vi "niFpgaFFTStreamingStateTransitionLogic.vi"(7 "reset":bool, 8 "output state in":enum8{"idle", "output"}(ring), 11 "process state in":enum8{"process", "idle"}(ring)) -> (0 "output state out":enum8{"idle", "output"}(ring), 2 "ready for input":bool, 3 "process state out":enum8{"process", "idle"}(ring))   [LabVIEW 2017]
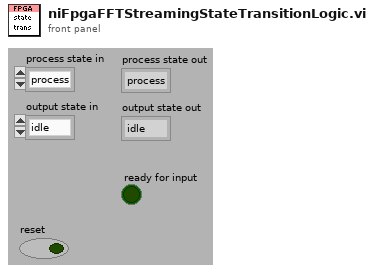
[diagram p1: front panel]
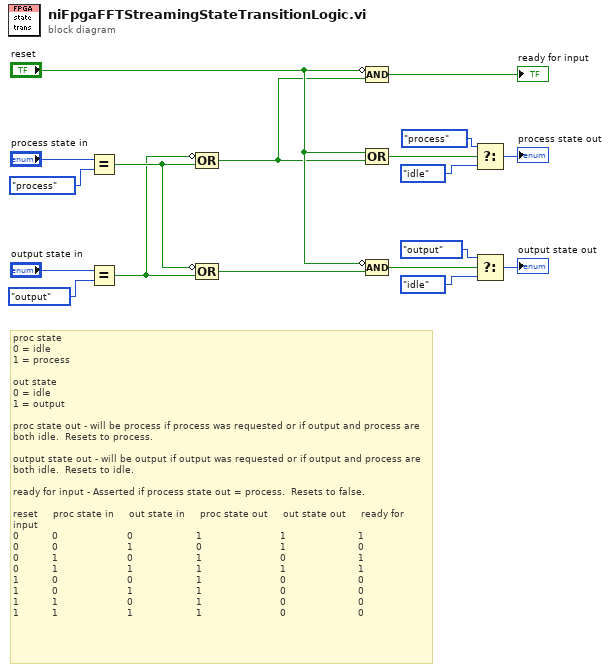
[diagram p0: block diagram]
diagram:
  # "proc state\n0 = idle\n1 = process\n\nout state\n0 = idle\n1 = output\n\nproc state out - will be process if process was requested or if output and process are both idle.  Resets to process.\n\noutput state out - will be output if output was requested or if output and process are both idle.  Resets to idle.\n\nready for input - Asserted if process state out = process.  Resets to false.\n\nreset     proc state in     out state in     proc state out     out state out     ready for input\n0           0                       0                     1                          1                        1 \n0           0                       1                     0                          1                        0\n0 \t\t        1                       0                     1                          0                        1\n0 \t\t        1                       1                     1                          1                        1\n1 \t\t        0                       0                     1                          0                        0\n1 \t\t        0                       1                     1                          0                        0\n1 \t\t        1                       0                     1                          0                        0\n1 \t\t        1                       1                     1                          0                        0"
  n1 = Equal?(x="process state in", y=enum8{"process", "idle"}."process") -> (x = y?=w5:bool)
  n2 = Equal?(x="output state in", y=enum8{"idle", "output"}."output" ("x")) -> (x = y?=w4:bool)
  n3 = Compound Arithmetic op=OR(invert w4, w5) -> (w3:bool)
  n4 = Compound Arithmetic op=OR(invert w5, w4) -> (w13:bool)
  n5 = Compound Arithmetic op=AND(invert "reset", w3) -> (→"ready for input":bool)
  n6 = Compound Arithmetic op=OR("reset", w3) -> (w7:bool)
  n7 = Compound Arithmetic op=AND(invert "reset", w13) -> (w9:bool)
  n8 = Select(t=enum8{"process", "idle"}."process", s=w7, f=enum8{"process", "idle"}."idle") -> (s? t:f=→"process state out":enum8{"process", "idle"})
  n9 = Select(t=enum8{"idle", "output"}."output", s=w9, f=enum8{"idle", "output"}."idle") -> (s? t:f=→"output state out":enum8{"idle", "output"})
